vi "analog dump viewer.vi"() -> ()   [LabVIEW 2018]
panel:
  in  "Stop Button":bool
  out "EOL Analog Trace Viewer":sgl[][](graph)
  in  "File":path
  # "v1.01"
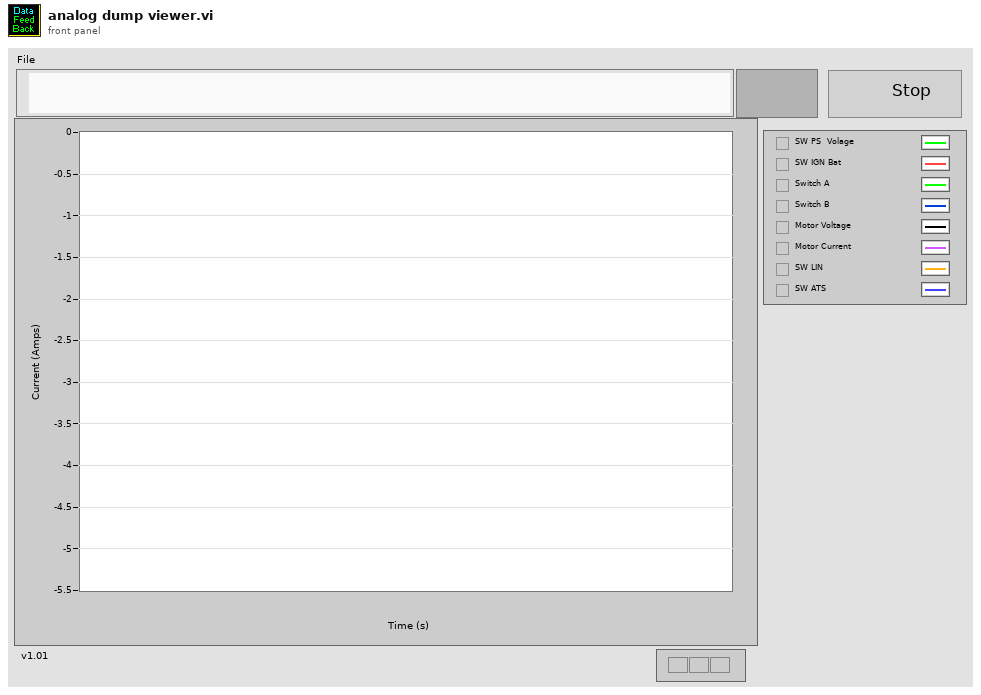
[diagram p1: front panel]
types:
  T1 = typedef "EOL Analog Input Control.ctl" = enum16{"SW PS  Volage", "SW IGN Bat", "Switch A", "Switch B", "Motor Voltage", "Motor Current", "SW LIN", "SW ATS"}
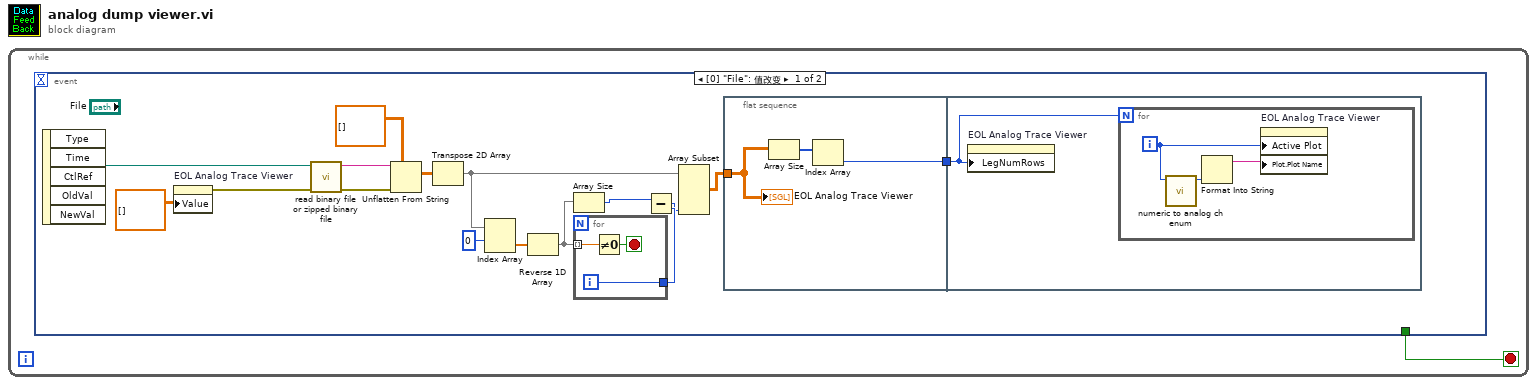
[diagram p0: block diagram]
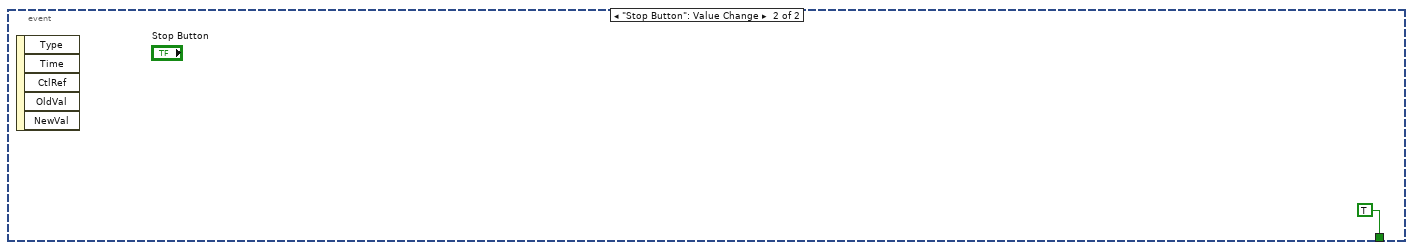
[diagram p2: hidden frame]
diagram:
  n1 = while {
    stop <- w1 stop-if-true
    n2 = event shown="[0] \"File\": 值改变" {
      selector: _ -> [_ _]
      dyn-events: _ -> [_ _]
      timeout: _ -> [_ _]
      tunnel: [_ TRUE] -> w1
      event "File": Value Change {
        n3 = event-data() -> ("NewVal"=w2:path)  [unwired: 1 in, 4 out]
        n4 = property on="EOL Analog Trace Viewer" class="WFGraph (严格)"("Value"=sgl[][] [] ("Motor Current Versus Time")) -> (error out=w7:errorcluster)  [unwired: 2 in, 1 out]
        n5 = call "read binary file or zipped binary file.vi"("error in"=w7, "File"=w2) -> ("error out"=w4:errorcluster, "data"=w5:string)  [unwired: 8 in]
        n6 = Unflatten From String(type=sgl[][] [], binary string=w5, error in (no error)=w4) -> (value=w3:sgl[][])  [unwired: 2 in, 2 out]
        n7 = Transpose 2D Array(2D array=w3) -> (transposed array=w13:sgl[][])
        n8 = Index Array(array=w13, index (row)=0) -> (element=w14:sgl[])  [unwired: 1 in]
        n9 = Reverse 1D Array(array=w14) -> (reversed array=w11:sgl[])
        n10 = Array Size(array=w11) -> (size(s)=w10:i32)
        n11 = for {
          tunnel: w11 -> [w20] mode=indexing
          tunnel: [w18] -> w9
          i -> [w18]
          stop <- w19 stop-if-true
          n12 = Not Equal To 0?(x=w20) -> (x != 0?=w19:bool)
        }
        n13 = Subtract(x=w10, y=w9) -> (x-y=w8:i32)
        n14 = Array Subset(array=w13, length (col)=w8) -> (w12:sgl[][])  [unwired: 3 in]
        n15 = flat-sequence {
          tunnel: w12 -> [w22]
          tunnel: [w21] -> w17
          tunnel: w17 -> [w24]
          frame #0 {
            n16 = Array Size(array=w22) -> (size(s)=w23:i32[])
            n17 = Index Array(array=w23) -> (element=w21:i32)  [unwired: 1 in]
            "EOL Analog Trace Viewer" <- w22
          }
          frame #1 {
            n18 = property on="EOL Analog Trace Viewer" class="WFGraph (严格)"("LegNumRows"=w24) -> ()  [unwired: 2 in, 2 out]
            n19 = for {
              N: w24 -> [_]
              i -> [w25]
              n20 = call "numeric to analog ch enum.vi"("Numeric"=w25) -> ("Analog Ch"=w27:T1)  [unwired: 10 in]
              n21 = Format Into String(w27) -> (resulting string=w26:string)  [unwired: 3 in, 1 out]
              n22 = property on="EOL Analog Trace Viewer" class="WFGraph (严格)"("Active Plot"=w25, "Plot.Plot Name"=w26) -> ()  [unwired: 2 in, 2 out]
            }
          }
        }
      }
      event "Stop Button": Value Change {
        n23 = event-data() -> ()  [unwired: 1 in, 5 out]
      }
    }
  }
